vi "20 Hatch Manipulator Bang Bang.vi"() -> ()   [LabVIEW 2018]
uses:
  <vilib>/Rock Robotics/WPI/Joystick/WPI_JoystickDeviceEnum.ctl
  <vilib>/Rock Robotics/SystemInterfaces/DIO/FPGA_DIOChannel.ctl
  <vilib>/Rock Robotics/SystemInterfaces/DIO/FPGA_DIOPWMChannel.ctl
  <vilib>/Rock Robotics/WPI/Encoder/WPI_EncoderType.ctl
  <vilib>/Rock Robotics/WPI/Switch/WPI_SwitchOpenLimit.vi
  <vilib>/Rock Robotics/WPI/MotorControl/WPI_MotorControlOpen SPARK.vi
  <vilib>/Rock Robotics/WPI/Counter/WPI_CounterDigitalInputToDigitalSource.vi
panel:
  in  "Hatch Backward Adjust Speed":dbl=0.4
  in  "Hatch Forward Adjust Speed":dbl=0.4
  in  "Hatch In Limit (X)":dbl
  in  "Hatch Out Limit (Y)":dbl
  in  "Hatch Backward Speed":dbl=0.5
  in  "Hatch Forward Speed":dbl=0.5
  in  "stop":bool
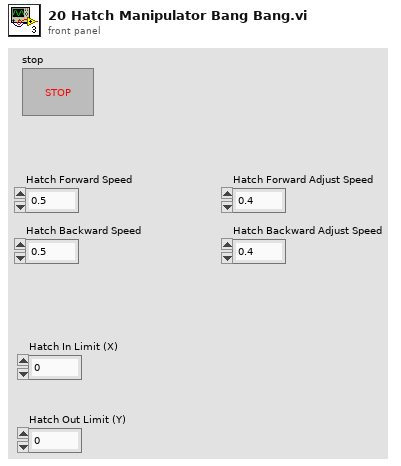
[diagram p1: front panel]
types:
  T1 = typedef "WPI_EncoderType.ctl" = enum16{"1x", "2x", "4x"}
  T2 = typedef "FPGA_DIOChannel.ctl" = enum8{"DIO 0", "DIO 1", "DIO 2", "DIO 3", "DIO 4", "DIO 5", "DIO 6", "DIO 7", "DIO 8", "DIO 9", "DIO MXP 0", "DIO MXP 1", "DIO MXP 2", "DIO MXP 3", "DIO MXP 4", "DIO MXP 5", "DIO MXP 6", "DIO MXP 7", "DIO MXP 8", "DIO MXP 9", "DIO MXP 10", "DIO MXP 11", "DIO MXP 12", "DIO MXP 13", "DIO MXP 14", "DIO MXP 15", "SPI Port CS1", "SPI Port CS2", "SPI Port CS3", "SPI Port MISO", "SPI Port MOSI", "Invalid"}
  T3 = typedef "FPGA_DIOPWMChannel.ctl" = enum8{"PWM 0", "PWM 1", "PWM 2", "PWM 3", "PWM 4", "PWM 5", "PWM 6", "PWM 7", "PWM 8", "PWM 9", "PWM MXP 0", "PWM MXP 1", "PWM MXP 2", "PWM MXP 3", "PWM MXP 4", "PWM MXP 5", "PWM MXP 6", "PWM MXP 7", "PWM MXP 8", "PWM MXP 9", "Invalid"}
  T4 = typedef "WPI_JoystickDeviceEnum.ctl" = enum16{"USB 0", "USB 1", "USB 2", "USB 3", "USB 4", "USB 5"}
  T5 = typedef "WPI_DigitalInputDevRef.ctl" = cluster{"DevStatus":errorcluster, "DIO Channel":T2}
  T6 = typedef "FPGA_CounterEncoderSourceConvertionLVSourceType.ctl" = cluster{"DevStatus":errorcluster, "AnalogTriggerMode?":bool, "DigitalMode":cluster{"DIO Channel":T7}, "AnalogTriggerMode":cluster{"AnalogTriggerIndex":T8, "OutputType":T9}}
  T7 = typedef "FPGA_DIODigitalSourceChannel.ctl" = enum8{"DIO 0", "DIO 1", "DIO 2", "DIO 3", "DIO 4", "DIO 5", "DIO 6", "DIO 7", "DIO 8", "DIO 9", "DIO MXP 0", "DIO MXP 1", "DIO MXP 2", "DIO MXP 3", "DIO MXP 4", "DIO MXP 5", "DIO MXP 6", "DIO MXP 7", "DIO MXP 8", "DIO MXP 9", "DIO MXP 10", "DIO MXP 11", "DIO MXP 12", "DIO MXP 13", "DIO MXP 14", "DIO MXP 15", "SPI Port CS1", "SPI Port CS2", "SPI Port CS3", "SPI Port MISO", "SPI Port MOSI", "Disabled"}
  T8 = typedef "FPGA_AnalogTriggerIndex.ctl" = enum8{"Trig 0", "Trig 1", "Trig 2", "Trig 3", "Trig 4", "Trig 5", "Trig 6", "Trig 7", "Invalid"}
  T9 = typedef "FPGA_AnalogTriggerOutType.ctl" = enum16{"InWindow", "TriggerState", "Rising", "Falling"}
  T10 = typedef "WPI_EncoderDevRef.ctl" = cluster{"DevStatus":errorcluster, "EncoderIndex":T11, "CounterIndex":T12, "DistancePerCount":dbl, "Decoding Type":T1}
  T11 = typedef "FPGA_EncoderIdx.ctl" = enum8{"Enc 0", "Enc 1", "Enc 2", "Enc 3", "Enc 4", "Enc 5", "Enc 6", "Enc 7", "Invalid"}
  T12 = typedef "FPGA_CounterCtrSystemIndex.ctl" = enum8{"Ctr 0", "Ctr 1", "Ctr 2", "Ctr 3", "Ctr 4", "Ctr 5", "Ctr 6", "Ctr 7", "Invalid"}
  T13 = typedef "WPI_SwitchDevRef.ctl" = cluster{"DevStatus":errorcluster, "DIO Channel":T2, "CntIndex":T12, "Normally Closed":bool}
  T14 = typedef "WPI_MotorControlDeviceRef.ctl" = cluster{"DeviceStatus":errorcluster, "Type":T15, "PWM":cluster{"PWM Channel":T3, "DeadBand":T16}, "CAN":cluster{"Device Number":u8, "SetOutput VI Ref":variant, "GetOutput VI Ref":variant, "Enable VI Ref":variant, "Disable VI Ref":variant, "Data":variant}, "Invert":bool, "DIO PWM":cluster{"PWM \"Enable\" Channel":T3, "DIOChannel":T2, "PWM Rate":dbl}}
  T15 = typedef "WPI_MotorControlType.ctl" = enum16{"PWM", "CAN", "DIO PWM"}
  T16 = typedef "WPI_PWMDeadband.ctl" = cluster{"Name":string, "maxPositivePwm":i32, "minPositivePwm":i32, "centerPwm":i32, "maxNegativePwm":i32, "minNegativePwm":i32, "angularRange":u16}
  T17 = typedef "WPI_JoystickDevRef.ctl" = cluster{"Device":T4}
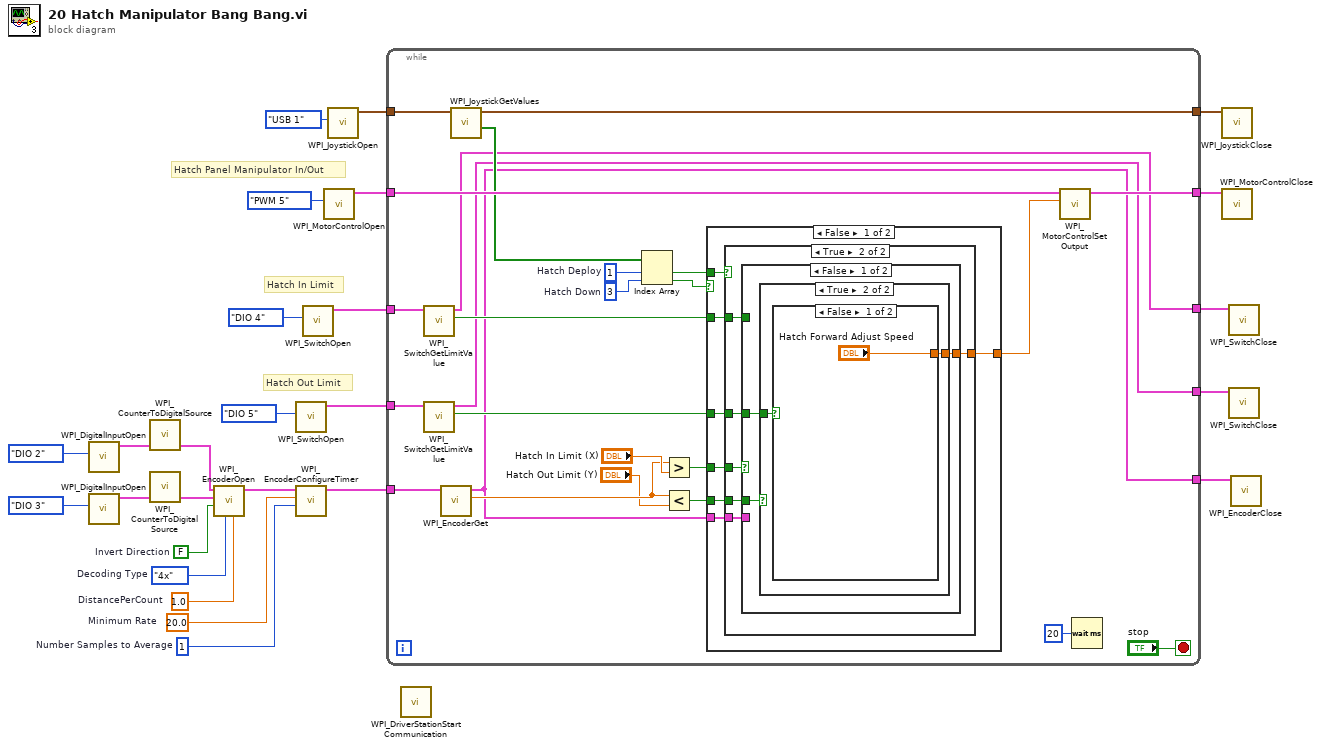
[diagram p0: block diagram]
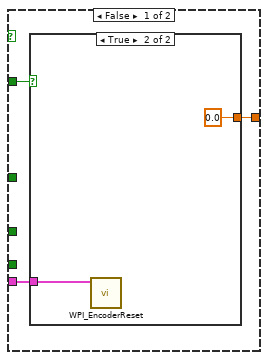
[diagram p2: hidden frame]
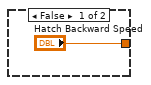
[diagram p3: hidden frame]
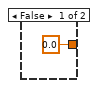
[diagram p4: hidden frame]
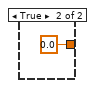
[diagram p5: hidden frame]
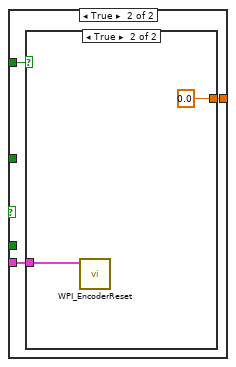
[diagram p6: hidden frame]
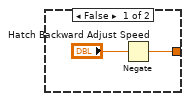
[diagram p7: hidden frame]
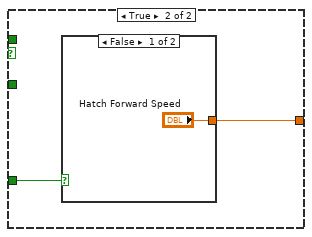
[diagram p8: hidden frame]
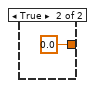
[diagram p9: hidden frame]
diagram:
  w3 = u8 1  # Number Samples to Average
  w4 = 20.0  # Minimum Rate
  w8 = 1.0  # DistancePerCount
  w7 = WPI_EncoderType."4x"  # Decoding Type
  w6 = FALSE  # Invert Direction
  # "Hatch Panel Manipulator In/Out"
  # "Hatch Out Limit"
  # "Hatch In Limit"
  n1 = call <vilib>:"WPI_DigitalInputOpen.vi"("DIO Channel"=FPGA_DIOChannel."DIO 2" ("A Channel")) -> ("DigitalInputDevRef"=w12:T5)  [unwired: 1 in, 9 out]
  n2 = call <vilib>:"WPI_DigitalInputOpen.vi"("DIO Channel"=FPGA_DIOChannel."DIO 3" ("B Channel")) -> ("DigitalInputDevRef"=w13:T5)  [unwired: 1 in, 9 out]
  n3 = call-poly <vilib>:"WPI_CounterToDigitalSource.vi"("DigitalInputDevRef"=w12) -> ("Digital Source"=w11:T6)  [unwired: 6 out]
  n4 = call-poly <vilib>:"WPI_CounterToDigitalSource.vi"("DigitalInputDevRef"=w13) -> ("Digital Source"=w14:T6)  [unwired: 6 out]
  n5 = call <vilib>:"WPI_EncoderOpen.vi"("DistancePerCount"=w8, "Decoding Type"=w7, "Invert Direction (False)"=w6, "BSource"=w14, "ASource"=w11) -> ("EncoderDevRef"=w5:T10)  [unwired: 3 in, 3 out]
  n6 = call-poly <vilib>:"WPI_SwitchOpen.vi"("DIO Channel"=FPGA_DIOChannel."DIO 5") -> ("SwitchDevRef"=w20:T13)  [unwired: 9 in, 1 out]
  n7 = call <vilib>:"WPI_EncoderConfigureTimer.vi"("Number Samples to Average"=w3, "Minimum Rate"=w4, "EncoderDevRef"=w5) -> ("EncoderDevRef"=w2:T10)  [unwired: 1 in, 7 out]
  n8 = call-poly <vilib>:"WPI_SwitchOpen.vi"("DIO Channel"=FPGA_DIOChannel."DIO 4") -> ("SwitchDevRef"=w21:T13)  [unwired: 9 in, 1 out]
  n9 = call-poly <vilib>:"WPI_MotorControlOpen.vi"("PWM Channel"=FPGA_DIOPWMChannel."PWM 5") -> ("MotorControlDeviceRef"=w18:T14)  [unwired: 9 in, 1 out]
  n10 = call <vilib>:"WPI_JoystickOpen.vi"("JoystickDevice"=WPI_JoystickDeviceEnum."USB 1") -> ("JoystickDevRef"=w25:T17)  [unwired: 10 in]
  n11 = while {
    tunnel: w25 -> [w49]
    tunnel: [w48] -> w24
    tunnel: w21 -> [w47]
    tunnel: w20 -> [w46]
    tunnel: w18 -> [w44]
    tunnel: [w45] -> w19
    tunnel: [w35] -> w16
    tunnel: [w34] -> w15
    tunnel: w2 -> [w33]
    tunnel: [w27] -> w1
    stop <- "stop" stop-if-true
    w41 = 3  # Hatch Down
    w42 = 1  # Hatch Deploy
    n12 = call <vilib>:"WPI_SwitchGetLimitValue.vi"("SwitchDevRef"=w47) -> ("Switch Pressed"=w39:bool, "SwitchDevRef"=w35:T13)  [unwired: 8 in, 1 out]
    n13 = call <vilib>:"WPI_SwitchGetLimitValue.vi"("SwitchDevRef"=w46) -> ("Switch Pressed"=w36:bool, "SwitchDevRef"=w34:T13)  [unwired: 8 in, 1 out]
    n14 = call <vilib>:"WPI_EncoderGet.vi"("EncoderDevRef"=w33) -> ("Distance"=w31:dbl, "EncoderDevRef"=w27:T10)  [unwired: 5 in, 4 out]
    n15 = call <vilib>:"WPI_JoystickGetValues.vi"("JoystickDevRef"=w49) -> ("Buttons"=w43:bool[], "JoystickDevRef"=w48:T17)  [unwired: 6 in, 3 out]
    n16 = Index Array(array=w43, index #1=w42, index #2=w41) -> (element #1=w40:bool, element #2=w37:bool)
    n17 = Greater?(x=w31, y="Hatch In Limit (X)") -> (0:w29:bool)
    n18 = Less?(x=w31, y="Hatch Out Limit (Y)") -> (x < y?=w28:bool)
    n19 = case shown="False" w37 {
      tunnel: w39 -> [w54 _]
      tunnel: [w57 w87] -> w38
      tunnel: w36 -> [w58 w86]
      tunnel: w40 -> [w56 _]
      tunnel: w29 -> [w55 _]
      tunnel: w28 -> [w53 _]
      tunnel: w27 -> [w52 _]
      frame False {
        n20 = case shown="True" w56 {
          tunnel: w58 -> [_ w66]
          tunnel: [w61 w70] -> w57
          tunnel: w55 -> [_ w69]
          tunnel: w54 -> [w60 w68]
          tunnel: w53 -> [_ w67]
          tunnel: w52 -> [w59 w65]
          frame False {
            n21 = case shown="True" w60 {
              tunnel: ["Hatch Backward Speed" 0.0 ("Wrist Out Speed")] -> w61
              tunnel: w59 -> [_ w63]
              frame False {
              }
              frame True {
                n22 = call <vilib>:"WPI_EncoderReset.vi"("EncoderDevRef"=w63) -> ()  [unwired: 9 in, 2 out]
              }
            }
          }
          frame True {
            n23 = case shown="False" w69 {
              tunnel: [w71 w81] -> w70
              tunnel: w68 -> [_ w80]
              tunnel: w67 -> [w73 _]
              tunnel: w66 -> [w72 _]
              tunnel: w65 -> [_ w79]
              frame False {
                n24 = case shown="True" w73 {
                  tunnel: w72 -> [_ w76]
                  tunnel: [0.0 ("Hatch Forward Adjust Speed") w75] -> w71
                  frame False {
                  }
                  frame True {
                    n25 = case shown="False" w76 {
                      tunnel: ["Hatch Forward Adjust Speed" 0.0 ("Hatch Forward Adjust Speed")] -> w75
                      frame False {
                      }
                      frame True {
                      }
                    }
                  }
                }
              }
              frame True {
                n26 = case shown="True" w80 {
                  tunnel: [w83 0.0] -> w81
                  tunnel: w79 -> [_ w84]
                  frame False {
                    n27 = Negate(x="Hatch Backward Adjust Speed") -> (-x=w83:dbl)
                  }
                  frame True {
                    n28 = call <vilib>:"WPI_EncoderReset.vi"("EncoderDevRef"=w84) -> ()  [unwired: 9 in, 2 out]
                  }
                }
              }
            }
          }
        }
      }
      frame True {
        n29 = case shown="False" w86 {
          tunnel: ["Hatch Forward Speed" 0.0] -> w87
          frame False {
          }
          frame True {
          }
        }
      }
    }
    n30 = call <vilib>:"WPI_MotorControlSetOutput.vi"("Output"=w38, "MotorControlDevRef"=w44) -> ("MotorControlDevRef"=w45:T14)  [unwired: 7 in, 2 out]
    n31 = Wait (ms)(milliseconds to wait=u32 20) -> ()  [unwired: 1 out]
  }
  n32 = call <vilib>:"WPI_DriverStationStart Communication.vi"() -> ()  [unwired: 12 in]
  n33 = call <vilib>:"WPI_JoystickClose.vi"("JoystickDevRef"=w24) -> ()  [unwired: 11 in]
  n34 = call <vilib>:"WPI_MotorControlClose.vi"("MotorControlDevRef"=w19) -> ()  [unwired: 10 in, 1 out]
  n35 = call <vilib>:"WPI_SwitchClose.vi"("SwitchDevRef"=w16) -> ()  [unwired: 10 in, 1 out]
  n36 = call <vilib>:"WPI_SwitchClose.vi"("SwitchDevRef"=w15) -> ()  [unwired: 10 in, 1 out]
  n37 = call <vilib>:"WPI_EncoderClose.vi"("EncoderDevRef"=w1) -> ()  [unwired: 10 in, 1 out]
